vi "Calculate Checksum.vi"(0 "Message":string, 11 "error in":errorcluster) -> (4 "MSG":string, 6 "CRC [String]":string, 8 "CRC [I32]":i32 format="%x", 15 "error out":errorcluster)   [LabVIEW 2018, in "Meerstetter Lib.lvlib" / "Meerstetter TEC.lvclass"]
doc: "This VI computes the CRC16 CCITT of any message. This implementation was derived from the C code provided by http://www.joegeluso.com/software/articles/ccitt.htm"
uses:
  Meerstetter TEC.lvclass
panel:
  # "POLY 1021"
  # "Initial Value = 0000"
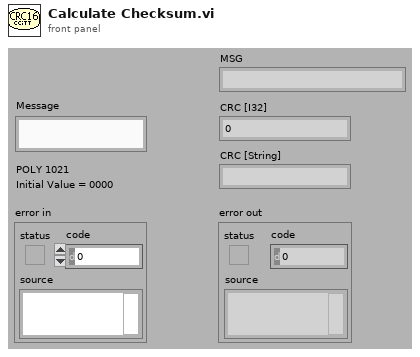
[diagram p1: front panel]
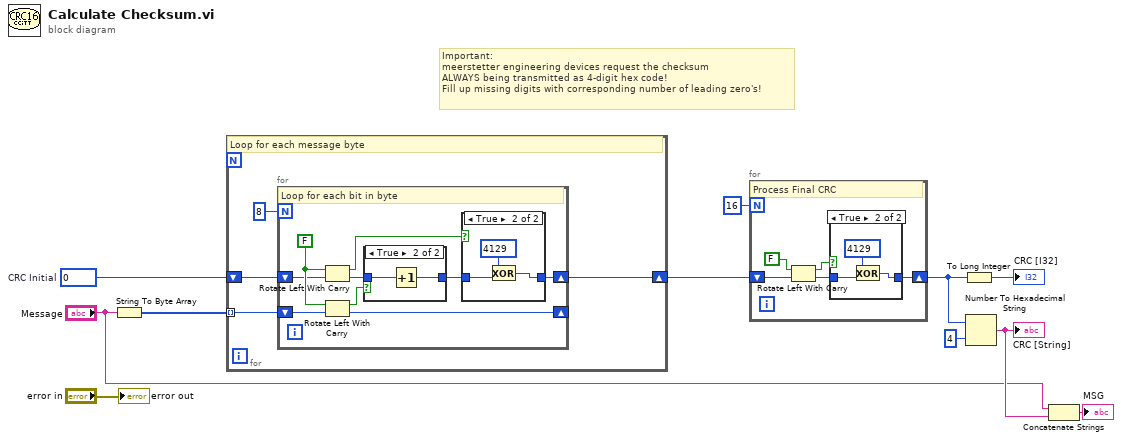
[diagram p0: block diagram]
diagram:
  w10 = u16 0  # CRC Initial
  # "Important:\nmeerstetter engineering devices request the checksum\nALWAYS being transmitted as 4-digit hex code!\nFill up missing digits with corresponding number of leading zero's!"
  n1 = String To Byte Array(string="Message") -> (unsigned byte array=w7:u8[])
  n2 = for "Loops for each message byte" {
    tunnel: w7 -> [w14] mode=indexing
    shift-right: [w12] -> w8
    shift-left: w10 -> [w13]
    # "Loop for each message byte"
    n3 = for "Loops for each bit in byte" {
      N: 8 -> [_]
      shift-right: [w19] -> _
      shift-left: w14 -> [w18]
      shift-right: [w16] -> w12
      shift-left: w13 -> [w17]
      w20 = FALSE ("carry")
      # "Loop for each bit in byte"
      n4 = Rotate Left With Carry(2:w17, 3:w20) -> (0:w23:u16, 1:w24:bool)
      n5 = Rotate Left With Carry(2:w18, 3:w20) -> (0:w19:u8, 1:w21:bool)
      n6 = case shown="True" w21 {
        tunnel: [w25 w26] -> w22
        tunnel: w23 -> [w25 w27]
        frame False {
        }
        frame True {
          n7 = Increment(x=w27) -> (x+1=w26:u16)
        }
      }
      n8 = case shown="True" w24 {
        tunnel: w22 -> [w28 w30]
        tunnel: [w28 w29] -> w16
        frame False {
        }
        frame True {
          n9 = Exclusive Or(1:w30, 2:u16 4129) -> (0:w29:u16)
        }
      }
    }
  }
  n10 = for {
    N: 16 -> [_]
    shift-right: [w34] -> w5
    shift-left: w8 -> [w33]
    # "Process Final CRC"
    n11 = Rotate Left With Carry(2:w33, 3:FALSE ("carry")) -> (0:w32:u16, 1:w36:bool)
    n12 = case shown="True" w36 {
      tunnel: w32 -> [w37 w38]
      tunnel: [w37 w39] -> w34
      frame False {
      }
      frame True {
        n13 = Exclusive Or(1:w38, 2:u16 4129) -> (0:w39:u16)
      }
    }
  }
  n14 = To Long Integer(number=w5) -> (32bit integer=→"CRC [I32]":i32)
  n15 = Number To Hexadecimal String(1:i16 4 ("width (-)"), 2:w5) -> (0:w3:string)
  "CRC [String]" <- w3
  n16 = Concatenate Strings("Message", w3) -> (→"MSG":string)
  "error out" <- "error in"
